vi "Rise and fall time evaluation.vi"(4 "sampling freq":dbl=1000.0 format="%#.3p", 6 "Upper_Thr":dbl=0.25 format="%#_13g", 7 "SiPM Waveform":waveform(dbl)[](array[waveform]), 8 "Fl":dbl=15.0 format="%#.3p", 9 "Fh":dbl=1.0 format="%#.3p", 10 "order":i32=2, 11 "V_thr":dbl) -> (0 "T3":dbl[](array[numeric]), 1 "T2":dbl[](array[numeric]), 2 "T1":dbl[](array[numeric]), 3 "Waveform Graph":dbl[][](graph))   [LabVIEW 2015]
uses:
  <vilib>/Analysis/3filter.llb/Butterworth Filter (DBL).vi
  <vilib>/Analysis/NI_AALBase.lvlib
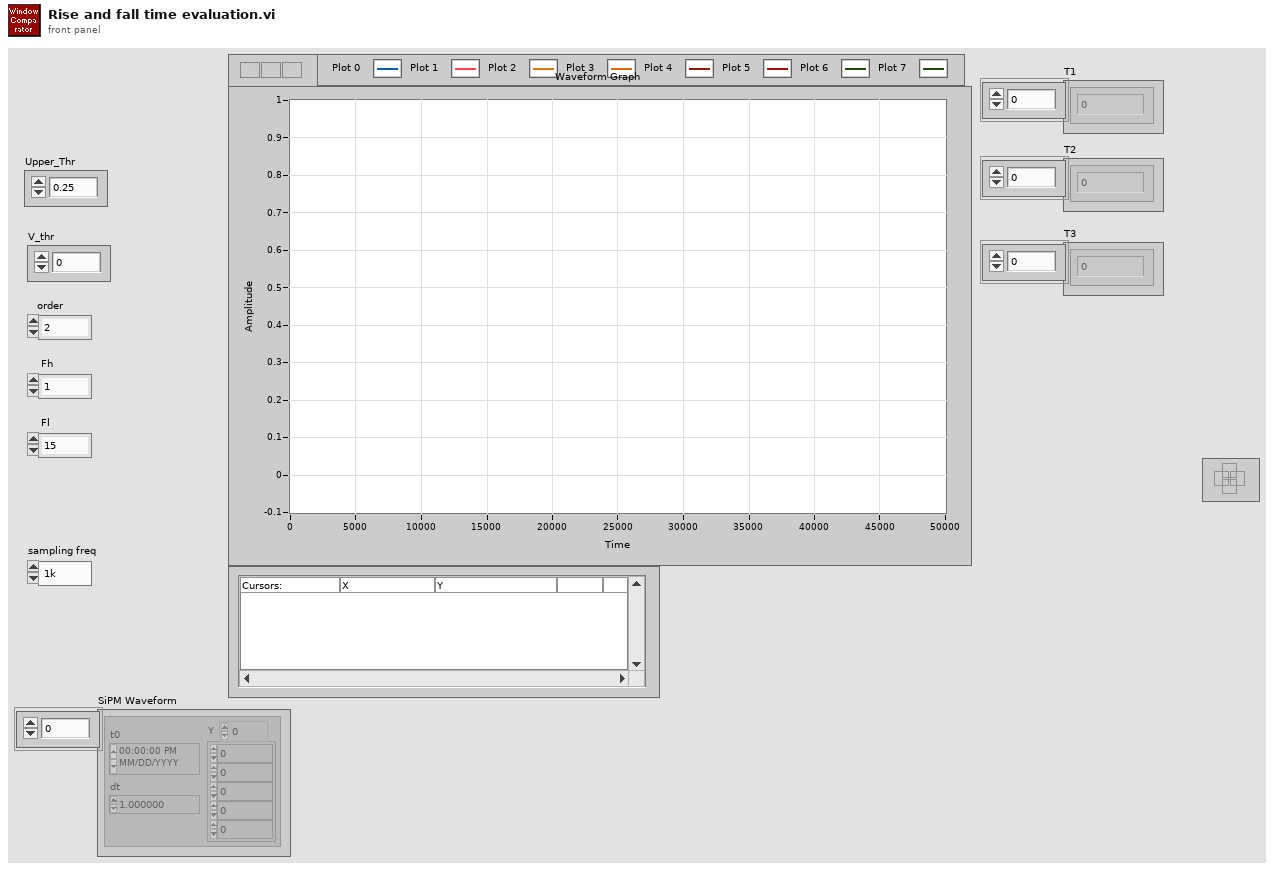
[diagram p1: front panel]
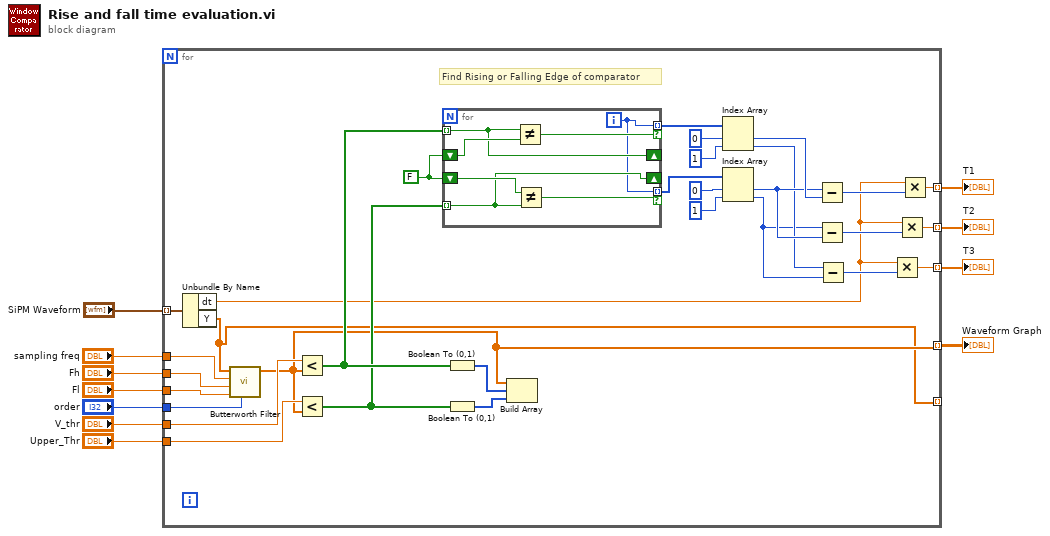
[diagram p0: block diagram]
diagram:
  n1 = for {
    tunnel: "order" -> [w42]
    tunnel: "Fh" -> [w41]
    tunnel: "Fl" -> [w40]
    tunnel: "sampling freq" -> [w39]
    tunnel: [w20] -> w7 mode=indexing
    tunnel: [w19] -> w6 mode=indexing
    tunnel: [w18] -> w5 mode=indexing
    tunnel: "SiPM Waveform" -> [w17] mode=indexing
    tunnel: "V_thr" -> [w16]
    tunnel: "Upper_Thr" -> [w15]
    tunnel: [w14] -> w1 mode=indexing
    tunnel: [w12] -> _ mode=indexing
    w34 = FALSE
    # "Find Rising or Falling Edge of comparator"
    n2 = Unbundle By Name(w17) -> ("dt"=w13:dbl, "Y"=w12:dbl[])
    n3 = call-poly <vilib>:"Butterworth Filter.vi"("order"=w42, "low cutoff freq: fl"=w40, "high cutoff freq: fh"=w41, "sampling freq: fs"=w39, "X"=w12) -> ("Filtered X"=w14:dbl[])  [unwired: 3 in, 1 out]
    n4 = Less?(x=w16, y=w14) -> (x < y?=w36:bool[])
    n5 = Less?(x=w15, y=w14) -> (x < y?=w35:bool[])
    n6 = for {
      tunnel: w36 -> [w48] mode=indexing
      shift-right: [w48] -> _
      shift-left: w34 -> [w49]
      tunnel: [w43] -> w33 mode=indexing if=w47
      shift-right: [w44] -> _
      shift-left: w34 -> [w46]
      tunnel: w35 -> [w44] mode=indexing
      tunnel: [w43] -> w28 mode=indexing if=w45
      i -> [w43]
      n7 = Not Equal?(x=w48, y=w49) -> (x != y?=w47:bool)
      n8 = Not Equal?(x=w46, y=w44) -> (x != y?=w45:bool)
    }
    n9 = Boolean To (0,1)(Boolean=w36) -> (0, 1=w37:i16[])
    n10 = Boolean To (0,1)(Boolean=w35) -> (0, 1=w38:i16[])
    n11 = Build Array(w14, w37, w38) -> ()  [unwired: 1 out]
    n12 = Index Array(array=w33, index #1=0 ("index"), index #2=1 ("index")) -> (element #1=w27:i32, element #2=w25:i32)
    n13 = Index Array(array=w28, index #1=0 ("index"), index #2=1 ("index")) -> (element #1=w26:i32, element #2=w24:i32)
    n14 = Subtract(x=w26, y=w27) -> (x-y=w23:i32)
    n15 = Subtract(x=w24, y=w26) -> (x-y=w22:i32)
    n16 = Subtract(x=w25, y=w24) -> (x-y=w21:i32)
    n17 = Multiply(x=w13, y=w21) -> (x*y=w18:dbl)
    n18 = Multiply(x=w13, y=w22) -> (x*y=w19:dbl)
    n19 = Multiply(x=w13, y=w23) -> (x*y=w20:dbl)
  }
  "T1" <- w7
  "T2" <- w6
  "T3" <- w5
  "Waveform Graph" <- w1
